vi "Tank_Feedback.vi"() -> (0 "Fill Density Meter":dbl format="%.3f", 4 "Tank D Level":dbl format="%.3f", 5 "Salt Saturator Level":dbl format="%.3f", 6 "Tank C Level":dbl format="%.3f", 7 "Tank B Level":dbl format="%.3f", 8 "Tank A Level":dbl format="%.3f", 9 "Comment":string)   [LabVIEW 2011]
uses:
  ADAM Client/Sub VIs/ADAM Controls/Address.ctl
panel:
  out "Sub3":cluster{"State":bool, "name":string}[](array[cluster])
  out "Sub2":cluster{"State":bool, "name":string}[](array[cluster])
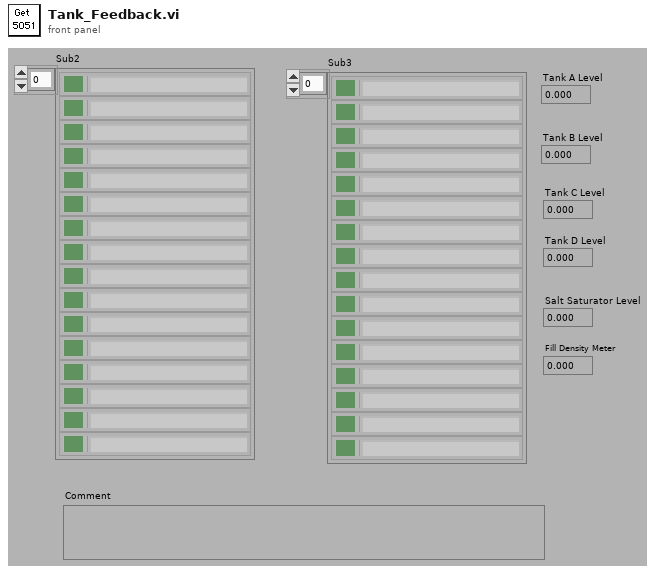
[diagram p1: front panel]
types:
  T1 = typedef "Address.ctl" = cluster{"Main":i32, "Ch.":i32, "Sub":i32, "Port Name":string}
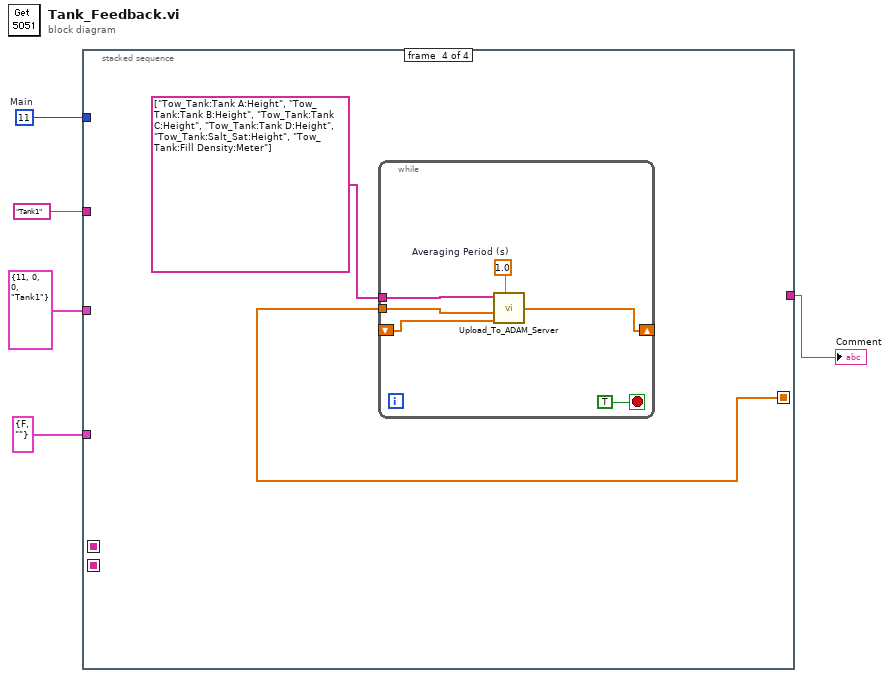
[diagram p0: block diagram]
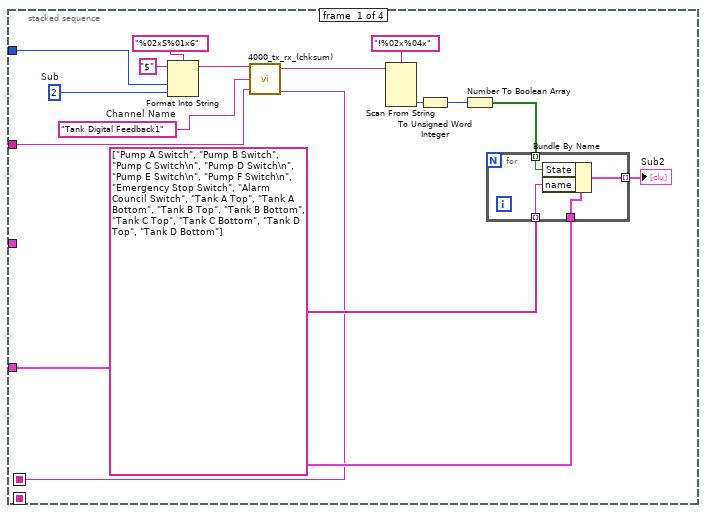
[diagram p2: hidden frame]
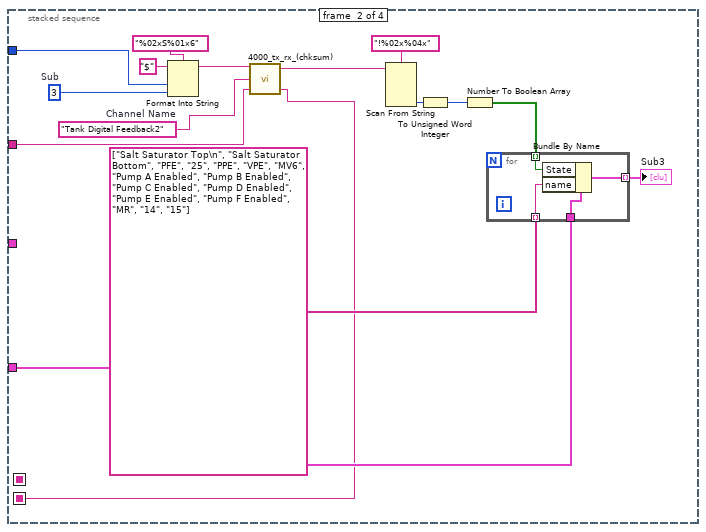
[diagram p3: hidden frame]
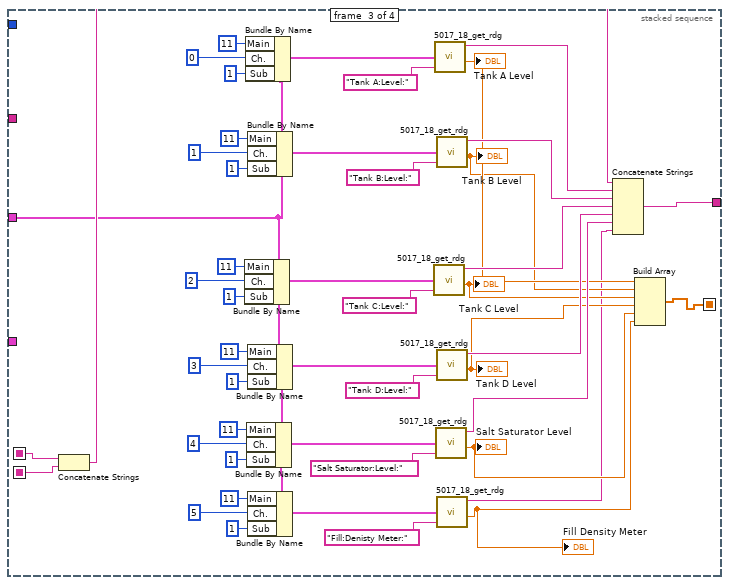
[diagram p4: hidden frame]
diagram:
  w4 = 11  # Main
  n1 = stacked-sequence {
    seq-local: [_ w26 _ _] -> [_ _ w67 _]
    seq-local: [w6 _ _ _] -> [_ _ w68 _]
    seq-local: [_ _ w54 _] -> [_ _ _ w95]
    tunnel: "Tank1" ("Port Name") -> [w14 w34 _ _]
    tunnel: w4 -> [w13 w33 _ _]
    tunnel: cluster{"State":bool, "name":string} {"State"=FALSE, "name"=""} ("Cluster") -> [w10 w30 _ _]
    tunnel: T1 {"Main"=11, "Ch."=0, "Sub"=0, "Port Name"="Tank1"} ("Address (all reqd.)") -> [_ _ w48 _]
    tunnel: [_ _ w60 _] -> w1
    frame #0 {
      w11 = "Tank Digital Feedback1"  # Channel Name
      w12 = 2  # Sub
      n2 = Format Into String(format string="%02xS%01x6", initial string="$", w13, w12) -> (resulting string=w19:string)  [unwired: 1 in, 1 out]
      n3 = call "4000_tx_rx_(chksum).vi"("Port Name"=w14, "Channel Name"=w11, "Write String"=w19) -> ("Comment out"=w6:string, "Read"=w18:string)  [unwired: 1 out]
      n4 = Scan From String(format string="!%02x%04x", input string=w18) -> (output 2=w15:i32)  [unwired: 2 in, 6 out]
      n5 = To Unsigned Word Integer(number=w15) -> (unsigned 16bit integer=w17:u16)
      n6 = Number To Boolean Array(number=w17) -> (Boolean array=w9:bool[])
      n7 = for {
        tunnel: w10 -> [w25]
        tunnel: w9 -> [w24] mode=indexing
        tunnel: string[] ["Pump A Switch", "Pump B Switch", "Pump C Switch\n", "Pump D Switch\n", "Pump E Switch\n", "Pump F Switch\n", "Emergency Stop Switch", "Alarm Council Switch", "Tank A Top", "Tank A Bottom", "Tank B Top", "Tank B Bottom", "Tank C Top", "Tank C Bottom", "Tank D Top", "Tank D Bottom"] -> [w23] mode=indexing
        tunnel: [w22] -> w7 mode=indexing
        n8 = Bundle By Name(cluster=w25, "State"=w24, "name"=w23) -> (w22:cluster{"State":bool, "name":string})
      }
      "Sub2" <- w7
    }
    frame #1 {
      w31 = "Tank Digital Feedback2"  # Channel Name
      w32 = 3  # Sub
      n9 = Format Into String(format string="%02xS%01x6", initial string="$", w33, w32) -> (resulting string=w39:string)  [unwired: 1 in, 1 out]
      n10 = call "4000_tx_rx_(chksum).vi"("Port Name"=w34, "Channel Name"=w31, "Write String"=w39) -> ("Comment out"=w26:string, "Read"=w38:string)  [unwired: 1 out]
      n11 = Scan From String(format string="!%02x%04x", input string=w38) -> (output 2=w35:i32)  [unwired: 2 in, 6 out]
      n12 = To Unsigned Word Integer(number=w35) -> (unsigned 16bit integer=w37:u16)
      n13 = Number To Boolean Array(number=w37) -> (Boolean array=w29:bool[])
      n14 = for {
        tunnel: w30 -> [w45]
        tunnel: w29 -> [w44] mode=indexing
        tunnel: string[] ["Salt Saturator Top\n", "Salt Saturator Bottom", "PFE", "25", "PPE", "VPE", "MV6", "Pump A Enabled", "Pump B Enabled", "Pump C Enabled", "Pump D Enabled", "Pump E Enabled", "Pump F Enabled", "MR", "14", "15"] -> [w43] mode=indexing
        tunnel: [w42] -> w27 mode=indexing
        n15 = Bundle By Name(cluster=w45, "State"=w44, "name"=w43) -> (w42:cluster{"State":bool, "name":string})
      }
      "Sub3" <- w27
    }
    frame #2 {
      n16 = Concatenate Strings(w68, w67) -> (w66:string)
      n17 = Bundle By Name(cluster=w48, "Main"=11, "Ch."=2, "Sub"=1) -> (w80:T1)
      n18 = Bundle By Name(cluster=w48, "Main"=11, "Ch."=0, "Sub"=1) -> (w90:T1)
      n19 = Bundle By Name(cluster=w48, "Main"=11, "Ch."=4, "Sub"=1) -> (w70:T1)
      n20 = Bundle By Name(cluster=w48, "Main"=11, "Ch."=1, "Sub"=1) -> (w87:T1)
      n21 = Bundle By Name(cluster=w48, "Main"=11, "Ch."=3, "Sub"=1) -> (w77:T1)
      n22 = Bundle By Name(cluster=w48, "Main"=11, "Ch."=5, "Sub"=1) -> (w52:T1)
      n23 = call "5017_18_get_rdg.vi"("Address (all reqd.)"=w80, "Channel Name"="Tank C:Level:") -> ("Comment"=w63:string, "Reading"=w57:dbl)  [unwired: 3 in]
      "Tank C Level" <- w57
      n24 = call "5017_18_get_rdg.vi"("Address (all reqd.)"=w90, "Channel Name"="Tank A:Level:") -> ("Comment"=w65:string, "Reading"=w59:dbl)  [unwired: 3 in]
      "Tank A Level" <- w59
      n25 = call "5017_18_get_rdg.vi"("Address (all reqd.)"=w70, "Channel Name"="Salt Saturator:Level:") -> ("Comment"=w61:string, "Reading"=w55:dbl)  [unwired: 3 in]
      "Salt Saturator Level" <- w55
      n26 = call "5017_18_get_rdg.vi"("Address (all reqd.)"=w87, "Channel Name"="Tank B:Level:") -> ("Comment"=w64:string, "Reading"=w58:dbl)  [unwired: 3 in]
      "Tank B Level" <- w58
      n27 = call "5017_18_get_rdg.vi"("Address (all reqd.)"=w77, "Channel Name"="Tank D:Level:") -> ("Comment"=w62:string, "Reading"=w56:dbl)  [unwired: 3 in]
      "Tank D Level" <- w56
      n28 = call "5017_18_get_rdg.vi"("Address (all reqd.)"=w52, "Channel Name"="Fill:Denisty Meter:") -> ("Comment"=w47:string, "Reading"=w46:dbl)  [unwired: 3 in]
      "Fill Density Meter" <- w46
      n29 = Concatenate Strings(w66, w65, w64, w63, w62, w61, w47) -> (w60:string)
      n30 = Build Array(w59, w58, w57, w56, w55, w46) -> (w54:dbl[])
    }
    frame #3 {
      n31 = while {
        shift-right: [w100] -> _
        shift-left: _ -> [w97]
        tunnel: w95 -> [w99]
        tunnel: string[] ["Tow_Tank:Tank A:Height", "Tow_Tank:Tank B:Height", "Tow_Tank:Tank C:Height", "Tow_Tank:Tank D:Height", "Tow_Tank:Salt_Sat:Height", "Tow_Tank:Fill Density:Meter"] -> [w96]
        stop <- TRUE stop-if-true
        w101 = 1.0  # Averaging Period (s)
        n32 = call "Upload_To_ADAM_Server.vi"("Averaging Period (s)"=w101, "Shift In"=w97, "Channel Values"=w99, "Channel Names"=w96) -> ("Shift Out"=w100:dbl[])  [unwired: 2 in]
      }
    }
  }
  "Comment" <- w1
